vi "amc_Send Message to Current Process.vi"(7 "Priority Message (F)":bool, 8 "error in (no error)":errorcluster, 10 "Message":T2, 11 "Message Queue in":T1) -> (0 "error out":errorcluster, 3 "Message Queue out":T1)   [LabVIEW 2011, in "ART2 Test Panel.lvlib" / "TLB_Dependencies.lvlib"]
uses:
  TLB_Dependencies.lvlib
  amc_Message.ctl
  Users/rkidagan/Dropbox/Atheros/ART2/Development/ART2 Test Panel/ART2 Test Panel/Components/Dependencies.llb/Keyed Array.ctl
  amc_Message Queue.ctl
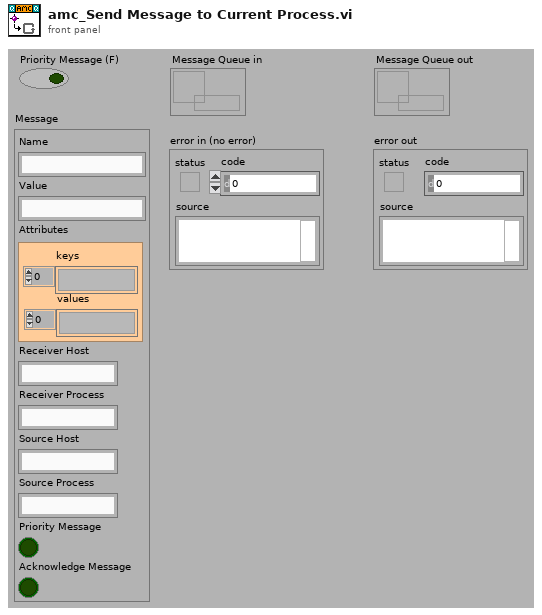
[diagram p1: front panel]
types:
  T1 = typedef "ART2 Test Panel.lvlib/TLB_Dependencies.lvlib/amc_Message Queue.ctl" = refnum<queue>
  T2 = typedef "ART2 Test Panel.lvlib/TLB_Dependencies.lvlib/amc_Message.ctl" = cluster{"Name":string, "Value":string, "Attributes":T3, "Receiver Host":string, "Receiver Process":string, "Source Host":string, "Source Process":string, "Priority Message":bool, "Acknowledge Message":bool}
  T3 = typedef "ART2 Test Panel.lvlib/TLB_Dependencies.lvlib/Keyed Array.ctl" = cluster{"keys":string[], "values":string[]}
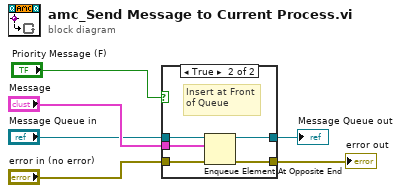
[diagram p0: block diagram]
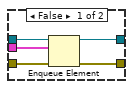
[diagram p2: hidden frame]
diagram:
  n1 = case shown="True" "Priority Message (F)" {
    tunnel: "Message Queue in" -> [w11 w13]
    tunnel: [w10 w14] -> w4
    tunnel: [w9 w15] -> w2
    tunnel: "error in (no error)" -> [w8 w16]
    tunnel: "Message" -> [w7 w12]
    frame False {
      n2 = Enqueue Element(queue=w11, element=w7, error in (no error)=w8) -> (queue out=w10:T1, error out=w9:errorcluster)  [unwired: 2 out]
    }
    frame True {
      # "Insert at Front\nof Queue"
      n3 = Enqueue Element At Opposite End(queue=w13, element=w12, error in (no error)=w16) -> (queue out=w14:T1, error out=w15:errorcluster)  [unwired: 2 out]
    }
  }
  "Message Queue out" <- w4
  "error out" <- w2
